vi "Do.vi"(8 "error in (no error)":errorcluster, 10 "Actor in":refnum<class "Actor.lvclass">, 11 "KIM101.lvlib:MoveBySteps Msg.lvclass":refnum<class "MoveBySteps Msg.lvclass">) -> (0 "error out":errorcluster, 2 "Actor out":refnum<class "Actor.lvclass">)   [LabVIEW 2023, in "MoveBySteps Msg.lvclass"]
doc: "This VI delivers the message to the actor by calling the appropriate method(s) on the actor."
uses:
  MoveBySteps Msg.lvclass
  9ef47adc-f318-494c-9b8b-6df3216d6863.vi
  KIM101/KIM101.lvclass
  C:/Program Files/National Instruments/LabVIEW 2023/vi.lib/ActorFramework/Message/Message.lvclass
  C:/Users/quantum/Downloads/SinglePhotonInterferometryUI-master/Libraries/KIM101_Actor/KIM101/KIM101 Messages/MoveBySteps Msg/MoveBySteps Msg.lvclass
  <vilib>/ActorFramework/Actor/Actor.lvclass
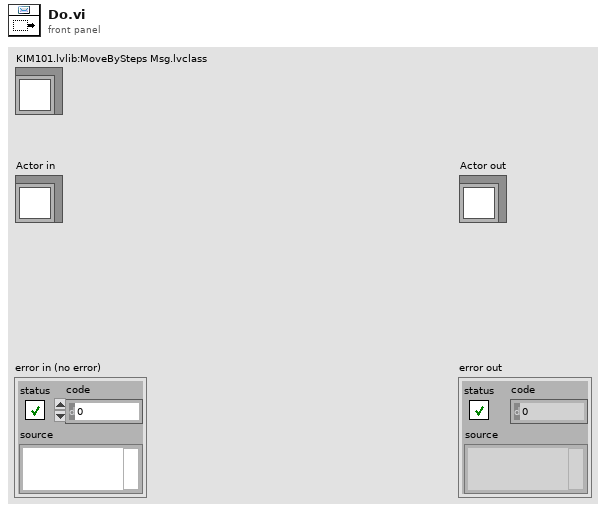
[diagram p1: front panel]
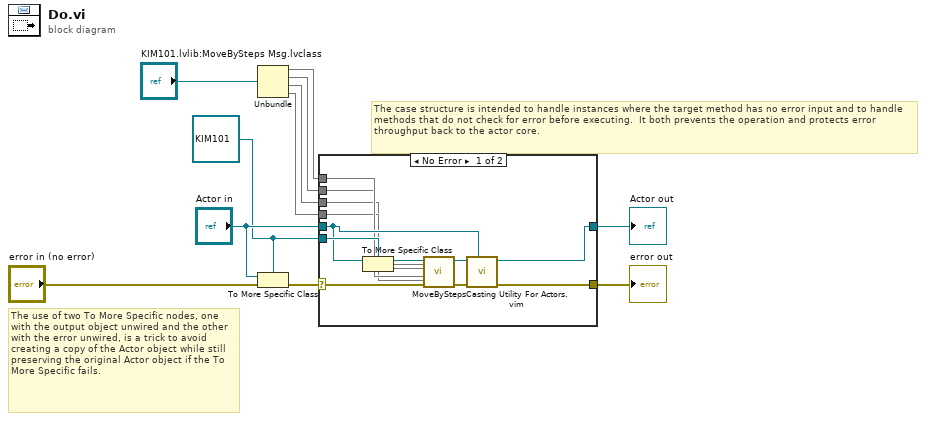
[diagram p0: block diagram]
diagram:
  w6 = refnum<class "KIM101.lvclass"> refnum ("Actor in")
  # "The use of two To More Specific nodes, one with the output object unwired and the other with the error unwired, is a trick to avoid creating a copy of the Actor object while still preserving the original Actor object if the To More Specific fails."
  # "The case structure is intended to handle instances where the target method has no error input and to handle methods that do not check for error before executing.  It both prevents the operation and protects error throughput back to the actor core."
  n1 = Unbundle("KIM101.lvlib:MoveBySteps Msg.lvclass") -> (w5, w4, w3, w2)
  n2 = To More Specific Class(target class=w6, reference="Actor in", error in="error in (no error)") -> (error out=w10:errorcluster)  [unwired: 1 out]
  n3 = case shown="No Error" w10 {
    selector: w10 -> [w23 w25]
    tunnel: [w17 w25] -> w9
    tunnel: [w18 w24] -> w8
    tunnel: "Actor in" -> [w20 w24]
    tunnel: w6 -> [w21 _]
    tunnel: w5 -> [w15 _]
    tunnel: w4 -> [w14 _]
    tunnel: w3 -> [w12 _]
    tunnel: w2 -> [w13 _]
    frame No Error {
      n4 = To More Specific Class(target class=w21, reference=w20) -> (specific class reference=w22:refnum<class "KIM101.lvclass">)  [unwired: 1 in, 1 out]
      n5 = call-dynamic "MoveBySteps.vi"("Polarity"=w12, "Direction"=w13, "error in (no error)"=w23, "Speed"=w14, "Steps"=w15, "TranslationStage in"=w22) -> ("error out"=w16:errorcluster, "TranslationStage out"=w19:refnum<class "KIM101.lvclass">)  [unwired: 4 in]
      n6 = call "Casting Utility For Actors.vim"("type"=w20, "error in (no error)"=w16, "Actor in"=w19) -> ("error out"=w17:errorcluster, "Actor out"=w18:refnum<class "Actor.lvclass">)  [unwired: 7 in]
    }
    frame Error {
      # "If type check fails, pass the original object out again."
    }
  }
  "error out" <- w9
  "Actor out" <- w8
